vi "自动缩进.vi"(8 "错误输入":errorcluster caption="错误输入（无错误）", 9 "扫描代码":i16, 11 "引用":refnum<k24>) -> (0 "错误输出":errorcluster, 3 "引用输出":refnum<k24>)   [LabVIEW 2020]
uses:
  D:/SuperPython-master/ScintillaNET.dll
  ScintillaNET.dll
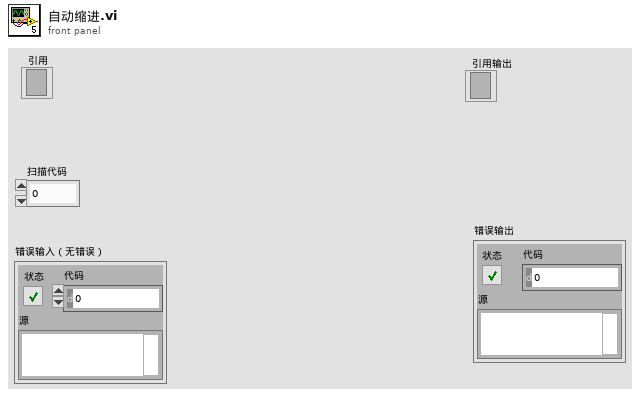
[diagram p1: front panel]
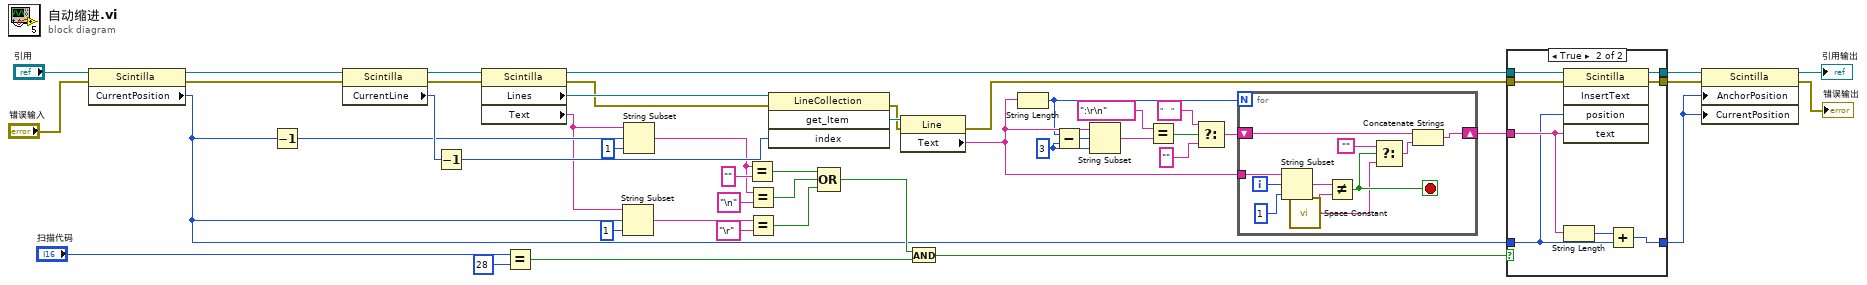
[diagram p0: block diagram]
diagram:
  w21 = 3 ("长度（剩余）")
  n1 = property class="Scintilla"(reference="引用", error in="错误输入") -> (reference out=w47:refnum<k24>, error out=w36:errorcluster, "CurrentPosition"=w4:i32)
  n2 = Decrement(x=w4) -> (x-1=w9:i32)
  n3 = property on="属性节点" class="Scintilla"(reference=w47, error in=w36) -> (reference out=w20:refnum<k24>, error out=w35:errorcluster, "CurrentLine"=w15:i32)
  n4 = Decrement(x=w15) -> (x-1=w44:i32)
  n5 = property class="Scintilla"(reference=w20, error in=w35) -> (reference out=w45:refnum<k24>, error out=w10:errorcluster, "Lines"=w19:refnum<k24>, "Text"=w5:string)
  n6 = Equal?(x="扫描代码", y=i16 28) -> (x = y?=w17:bool)
  n7 = String Subset(string=w5, offset (0)=w4, length (rest)=1 ("长度（剩余）")) -> (substring=w2:string)
  n8 = String Subset(string=w5, offset (0)=w9, length (rest)=1 ("长度（剩余）")) -> (substring=w7:string)
  n9 = Equal?(x=w7, y="") -> (x = y?=w14:bool)
  n10 = Equal?(x=w7, y="\n") -> (x = y?=w11:bool)
  n11 = Equal?(x=w2, y="\r") -> (x = y?=w1:bool)
  n12 = invoke class="LineCollection" method="get_Item"(reference=w19, error in=w10, "index"=w44) -> (error out=w34:errorcluster, "get_Item"=w46:refnum<k24>)  [unwired: 1 in, 2 out]
  n13 = Compound Arithmetic op=OR ("复合运算")(w14, w11, w1) -> (w13:bool)
  n14 = property class="Line"(reference=w46, error in=w34) -> (error out=w33:errorcluster, "Text"=w30:string)  [unwired: 1 out]
  n15 = And(x=w13, y=w17) -> (x .and. y?=w16:bool)
  n16 = String Length(string=w30) -> (length=w23:i32)
  n17 = Subtract(x=w23, y=w21) -> (x-y=w22:i32)
  n18 = String Subset(string=w30, offset (0)=w22, length (rest)=w21) -> (substring=w29:string)
  n19 = Equal?(x=":\r\n", y=w29) -> (x = y?=w27:bool)
  n20 = Select(t="    ", s=w27, f="") -> (s? t:f=w26:string)
  n21 = for {
    N: w23 -> [_]
    tunnel: w30 -> [w58]
    shift-right: [w55] -> w41
    shift-left: w26 -> [w54]
    i -> [w56]
    stop <- w53 stop-if-true
    n22 = String Subset(string=w58, offset (0)=w56, length (rest)=1 ("长度（剩余）")) -> (substring=w51:string)
    n23 = call <vilib>:"Space Constant.vi"() -> ("String"=w49:string)
    n24 = Not Equal?(x=w51, y=w49) -> (x != y?=w53:bool)
    n25 = Select(t="", s=w53, f=w49) -> (s? t:f=w52:string)
    n26 = Concatenate Strings(w54, w52) -> (w55:string)
  }
  n27 = case shown="True" w16 {
    tunnel: [w61 w69] -> w40
    tunnel: w4 -> [w60 w65]
    tunnel: w45 -> [w61 w68]
    tunnel: w41 -> [_ w67]
    tunnel: [w60 w64] -> w38
    tunnel: w33 -> [w59 w63]
    tunnel: [w59 w62] -> w32
    frame False {
    }
    frame True {
      n28 = invoke on="调用节点" class="Scintilla" method="InsertText"(reference=w68, error in=w63, "position"=w65, "text"=w67) -> (reference out=w69:refnum<k24>, error out=w62:errorcluster)  [unwired: 1 in, 3 out]
      n29 = String Length(string=w67) -> (length=w66:i32)
      n30 = Add(x=w66, y=w65) -> (x+y=w64:i32)
    }
  }
  n31 = property on="属性节点" class="Scintilla"(reference=w40, error in=w32, "AnchorPosition"=w38, "CurrentPosition"=w38) -> (reference out=→"引用输出":refnum<k24>, error out=→"错误输出":errorcluster)
